vi "Byte Array to unsigned Int.vi"(1 "buffer in":u8[](array[numeric])) -> (0 "unsigned int out":u32)   [LabVIEW 2014]
doc: "This VI takes byte array and going from end to beginning is pushing these bytes into result unsinged int, so they all will be in one 32b variable in reversed order."
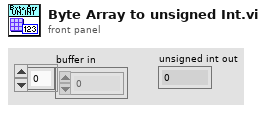
[diagram p1: front panel]
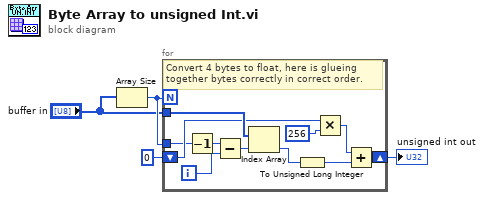
[diagram p0: block diagram]
diagram:
  n1 = Array Size(array="buffer in") -> (size(s)=w4:i32)
  n2 = for {
    N: w4 -> [_]
    tunnel: "buffer in" -> [w15]
    shift-right: [w10] -> w1
    shift-left: u32 0 ("element") -> [w14]
    tunnel: w4 -> [w9]
    i -> [w8]
    # "Convert 4 bytes to float, here is glueing together bytes correctly in correct order."
    n3 = Decrement(x=w9) -> (x-1=w7:i32)
    n4 = Subtract(x=w7, y=w8) -> (x-y=w6:i32)
    n5 = Index Array(array=w15, index=w6) -> (element=w11:u8)
    n6 = To Unsigned Long Integer(number=w11) -> (unsigned 32bit integer=w5:u32)
    n7 = Multiply(x=w14, y=u32 256) -> (x*y=w12:u32)
    n8 = Add(x=w12, y=w5) -> (x+y=w10:u32)
  }
  "unsigned int out" <- w1
